vi "FPGA_Control.vi"() -> ()   [LabVIEW 2022 SP3]
uses:
  <vilib>/regexp/Match Regular Expression.xnode
panel:
  in  "Pulse Configuration":T1(tab)
  out "Detected COM Port":string
  out "DLP-232PC Found":bool
  in  "Start Search":bool
  out "ASCII string":string[](array[string])
  out "Digital Outputs":bool[](array[boolean])
  out "High1 Time(ns)":dbl
  in  "Set High1 Time":i16(knob) min=0 step=1 scale=0.0..255.0
  out "ASCII string 2":string[](array[string])
  out "Digital Outputs 2":bool[](array[boolean])
  in  "Set High2 Time":i8(knob) scale=0.0..31.0
  out "High2 Time(ns)":dbl
  in  "Send Pulse":bool
  out "Pulse Sent":bool
  out "VISA resource name out":refnum<visa-resource-name>
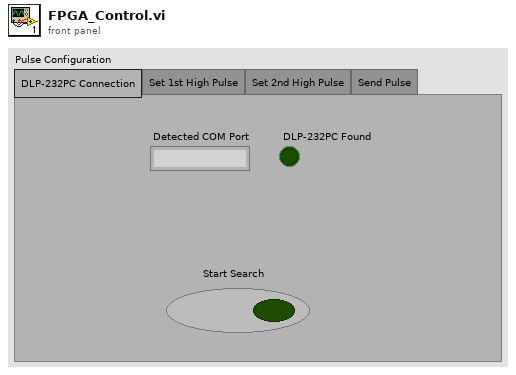
[diagram p1: front panel]
types:
  T1 = enum32{"DLP-232PC Connection", "Set 1st High Pulse", "Set 2nd High Pulse", "Send Pulse"}
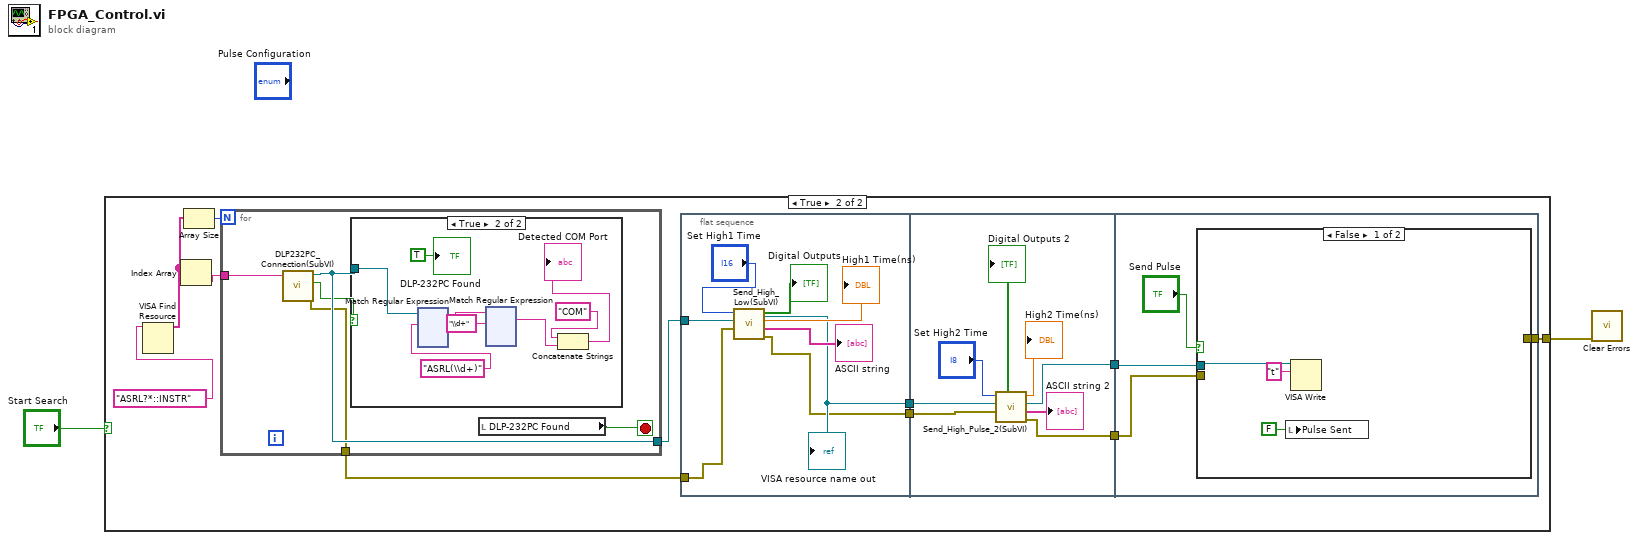
[diagram p0: block diagram]
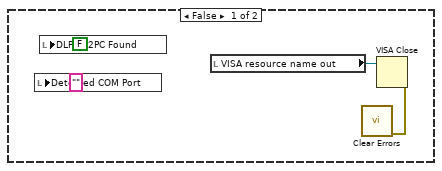
[diagram p2: hidden frame]
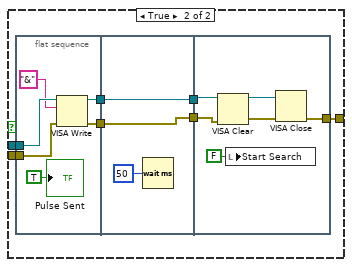
[diagram p3: hidden frame]
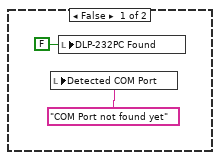
[diagram p4: hidden frame]
diagram:
  n1 = case shown="True" "Start Search" {
    tunnel: [_ w7] -> w1
    frame False {
      n2 = local write "Detected COM Port"("" ("Detected COM Port")) -> ()
      n3 = local write "DLP-232PC Found"(FALSE ("DLP-232PC Found")) -> ()
      n4 = local read "VISA resource name out"() -> (w3:refnum<visa-resource-name>)
      n5 = VISA Close(VISA resource name=w3) -> (error out=w4:errorcluster)  [unwired: 1 in]
      n6 = call <vilib>:"Clear Errors.vi"("error in (no error)"=w4) -> ()  [unwired: 5 in, 2 out]
    }
    frame True {
      n7 = VISA Find Resource(11:"ASRL?*::INSTR" ("expression (\"?*\")")) -> (3:w15:string[])  [unwired: 2 in, 2 out]
      n8 = Index Array(array=w15) -> (element=w14:string)  [unwired: 1 in]
      n9 = Array Size(array=w15) -> (size(s)=w16:i32)
      n10 = for {
        N: w16 -> [_]
        tunnel: w14 -> [w64]
        tunnel: [w66] -> w13
        tunnel: [w63] -> w8
        stop <- w67 stop-if-true
        n11 = call "DLP232PC_Connection(SubVI).vi"("String"=w64) -> ("error out"=w63:errorcluster, "Boolean"=w65:bool, "VISA Refnum out"=w66:refnum<visa-resource-name>)  [unwired: 8 in]
        n12 = case shown="True" w65 {
          tunnel: w66 -> [_ w74]
          frame False {
            n13 = local write "Detected COM Port"("COM Port not found yet" ("Detected COM Port")) -> ()
            n14 = local write "DLP-232PC Found"(FALSE ("DLP-232PC Found")) -> ()
          }
          frame True {
            n15 = xnode "Match Regular Expression"("input string"=w74, "regular expression"="ASRL(\\d+)") -> ("whole match"=w72:string)  [unwired: 4 in, 4 out]
            n16 = xnode "Match Regular Expression"("input string"=w72, "regular expression"="\\d+") -> ("whole match"=w70:string)  [unwired: 4 in, 4 out]
            n17 = Concatenate Strings("COM" ("string"), w70) -> (→"Detected COM Port":string)
            "DLP-232PC Found" <- TRUE ("DLP-232PC Found")
          }
        }
        n18 = local read "DLP-232PC Found"() -> (w67:bool)
      }
      n19 = flat-sequence {
        tunnel: w13 -> [w22]
        tunnel: [w20] -> w12
        tunnel: [w19] -> w9
        tunnel: w8 -> [w18]
        tunnel: w12 -> [w33]
        tunnel: [w28] -> w11
        tunnel: [w27] -> w10
        tunnel: w9 -> [w26]
        tunnel: w11 -> [w36]
        tunnel: w10 -> [w35]
        tunnel: [w34] -> w7
        frame #0 {
          n20 = call "Send_High_Low(SubVI).vi"("error in (no error)"=w18, "VISA resource name"=w22, "Set High1 Time"="Set High1 Time") -> ("error out"=w19:errorcluster, "ASCII string"=→"ASCII string":string[], "High1 Time(ns)"=→"High1 Time(ns)":dbl, "Digital Outputs"=→"Digital Outputs":bool[], "VISA resource name out"=w20:refnum<visa-resource-name>)  [unwired: 3 in, 1 out]
          "VISA resource name out" <- w20
        }
        frame #1 {
          n21 = call "Send_High_Pulse_2(SubVI).vi"("error in (no error)"=w26, "VISA resource name"=w33, "Set High2 Time"="Set High2 Time") -> ("error out"=w27:errorcluster, "ASCII string"=→"ASCII string 2":string[], "VISA resource name out"=w28:refnum<visa-resource-name>, "High2 Time(ns)"=→"High2 Time(ns)":dbl, "Digital Outputs"=→"Digital Outputs 2":bool[])  [unwired: 3 in, 1 out]
        }
        frame #2 {
          n22 = case shown="False" "Send Pulse" {
            tunnel: w36 -> [w40 w47]
            tunnel: w35 -> [_ w45]
            tunnel: [_ w41] -> w34
            frame False {
              n23 = local write "Pulse Sent"(FALSE ("Pulse Sent")) -> ()
              n24 = VISA Write(VISA resource name=w40, write buffer="t") -> ()  [unwired: 1 in, 3 out]
            }
            frame True {
              n25 = flat-sequence {
                tunnel: w47 -> [w53]
                tunnel: [w50] -> w46
                tunnel: w45 -> [w49]
                tunnel: [w48] -> w42
                tunnel: w46 -> [w56]
                tunnel: [w56] -> w44
                tunnel: [w54] -> w43
                tunnel: w42 -> [w54]
                tunnel: w44 -> [w59]
                tunnel: w43 -> [w60]
                tunnel: [w61] -> w41
                frame #0 {
                  n26 = VISA Write(VISA resource name=w53, write buffer="&", error in (no error)=w49) -> (VISA resource name out=w48:refnum<visa-resource-name>, error out=w50:errorcluster)  [unwired: 1 out]
                  "Pulse Sent" <- TRUE ("Pulse Sent")
                }
                frame #1 {
                  n27 = Wait (ms)(milliseconds to wait=u32 50) -> ()  [unwired: 1 out]
                }
                frame #2 {
                  n28 = VISA Clear(VISA resource name=w60, error in (no error)=w59) -> (VISA resource name out=w57:refnum<visa-resource-name>, error out=w58:errorcluster)
                  n29 = local write "Start Search"(FALSE ("Start Search")) -> ()
                  n30 = VISA Close(VISA resource name=w57, error in (no error)=w58) -> (error out=w61:errorcluster)
                }
              }
            }
          }
        }
      }
    }
  }
  n31 = call <vilib>:"Clear Errors.vi"("error in (no error)"=w1) -> ()  [unwired: 5 in, 2 out]
